vi "Post-Build Action.vi"(5 "Files Generated by Build":path[](array[path]), 6 "Top Level/Always Included VIs":path[](array[path]), 7 "Destination Path":path, 8 "error in (no error)":errorcluster, 9 "Target Name":string, 10 "Build Specification Name":string, 11 "Project Path":path) -> (0 "error out":errorcluster)   [LabVIEW 2019, in "Tools.lvlib"]
doc: "This VI deletes CreateVerificationFile(Automatic).vi from compiled application. More post-build actions can be added if necessary."
uses:
  Tools.lvlib
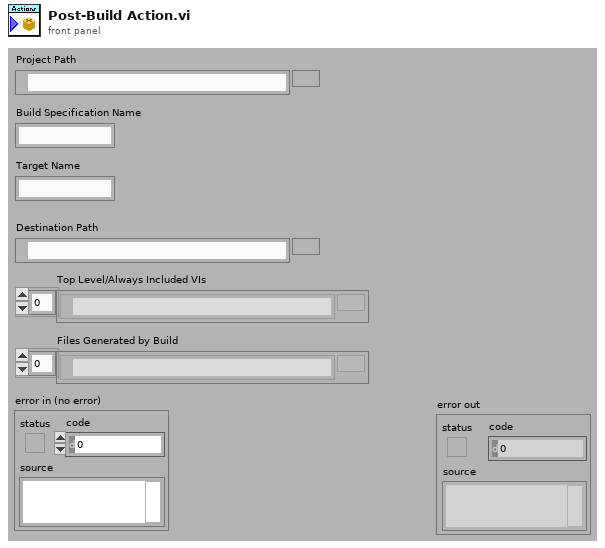
[diagram p1: front panel]
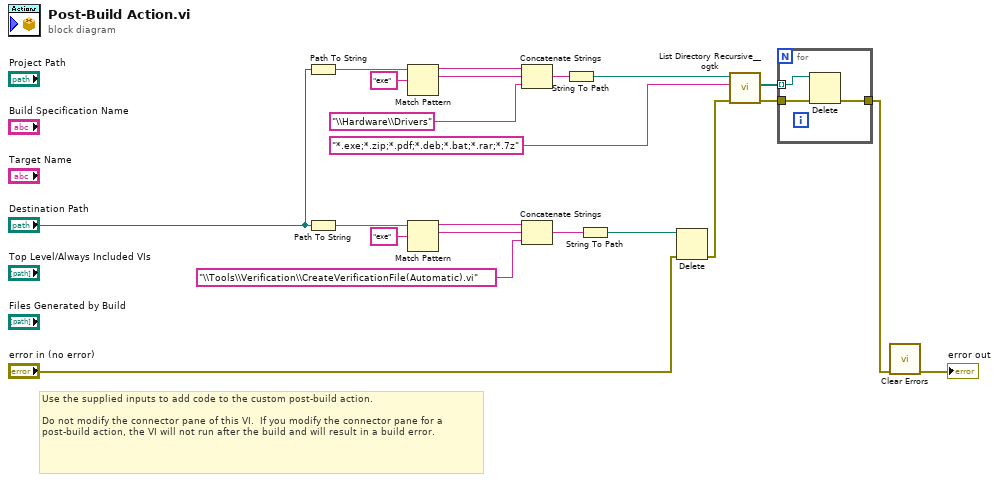
[diagram p0: block diagram]
diagram:
  # "Use the supplied inputs to add code to the custom post-build action.\n\nDo not modify the connector pane of this VI.  If you modify the connector pane for a post-build action, the VI will not run after the build and will result in a build error."
  n1 = Path To String(path="Destination Path") -> (string=w13:string)
  n2 = Path To String(path="Destination Path") -> (string=w22:string)
  n3 = Match Pattern(string=w13, regular expression="exe") -> (before substring=w11:string, match substring=w10:string)  [unwired: 1 in, 2 out]
  n4 = Match Pattern(string=w22, regular expression="exe") -> (before substring=w20:string, match substring=w19:string)  [unwired: 1 in, 2 out]
  n5 = Concatenate Strings(w11, w10, "\\Hardware\\Drivers" ("string")) -> (w8:string)
  n6 = Concatenate Strings(w20, w19, "\\Tools\\Verification\\CreateVerificationFile(Automatic).vi" ("string")) -> (w17:string)
  n7 = String To Path(string=w8) -> (path=w6:path)
  n8 = String To Path(string=w17) -> (path=w16:path)
  n9 = Delete(path (use dialog)=w16, error in="error in (no error)") -> (error out=w5:errorcluster)  [unwired: 3 in, 2 out]
  n10 = call <userlib>:"List Directory Recursive__ogtk.vi"("error in (no error)"=w5, "pattern"="*.exe;*.zip;*.pdf;*.deb;*.bat;*.rar;*.7z", "Path"=w6) -> ("error out"=w3:errorcluster, "file paths"=w4:path[])  [unwired: 5 in, 2 out]
  n11 = for {
    tunnel: w4 -> [w25] mode=indexing
    tunnel: w3 -> [w24]
    tunnel: [w23] -> w2
    n12 = Delete(path (use dialog)=w25, error in=w24) -> (error out=w23:errorcluster)  [unwired: 3 in, 2 out]
  }
  n13 = call <vilib>:"Clear Errors.vi"("error in (no error)"=w2) -> ("error out"=→"error out":errorcluster)  [unwired: 5 in, 1 out]
